vi "Begin.vi"() -> (1 "CameraDevRef":T1)   [LabVIEW 2011]
doc: "Called before other user functions, this VI is expected to open initial I/O refnums, load in file data, and do all program initialization. Notice that the <B>error out</B> terminal is simply used for data flow. Wiring it to other structures or subVIs ensures that this VI runs first."
uses:
  <vilib>/Rock Robotics/WPI/Camera/WPI_CameraDevRef.ctl
  <vilib>/Rock Robotics/SystemInterfaces/DIO/FPGA_DIOPWMChannel.ctl
  <vilib>/Rock Robotics/WPI/Joystick/WPI_JoystickDeviceEnum.ctl
  <vilib>/Rock Robotics/SystemInterfaces/AI/FPGA_AIChannel.ctl
  <vilib>/Rock Robotics/SystemInterfaces/DIO/FPGA_DIORelayChannel.ctl
  <vilib>/Rock Robotics/SystemInterfaces/DIO/FPGA_DIOChannel.ctl
  <vilib>/Rock Robotics/SystemInterfaces/AI/FPGA_AIGyroChannel.ctl
  <vilib>/Rock Robotics/WPI/MotorControl/WPI_MotorControlOpen Victor.vi
  <vilib>/Rock Robotics/WPI/MotorControl/WPI_MotorControlOpen Jaguar.vi
  Robot Global Data.vi
  <vilib>/Utility/file.llb/Read From Spreadsheet File (DBL).vi
  <vilib>/Rock Robotics/WPI/Relay/WPI_RelayDirection.ctl
  <vilib>/Rock Robotics/SystemInterfaces/Typedef/FPGA_TypedefDigitalModule.ctl
  <vilib>/Rock Robotics/WPI/Counter/WPI_CounterDigitalInputToDigitalSource.vi
  <vilib>/Rock Robotics/WPI/Encoder/WPI_EncoderType.ctl
  <vilib>/Rock Robotics/SystemInterfaces/Typedef/FPGA_TypedefAnalogModule.ctl
panel:
  out "Path and file":string
  in  "Balls In Robot At Start":dbl
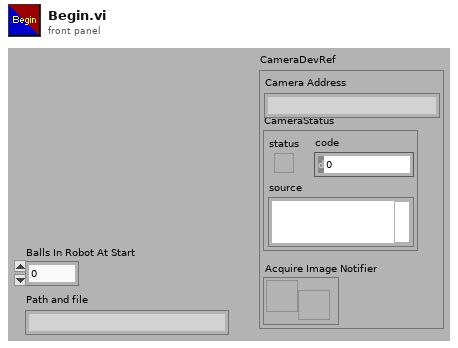
[diagram p1: front panel]
types:
  T1 = typedef "WPI_CameraDevRef.ctl" = cluster{"Camera Address":string, "CameraStatus":errorcluster, "Acquire Image Notifier":refnum<notifier>}
  T2 = typedef "FPGA_AIGyroChannel.ctl" = enum8{"AI 1", "AI 2", "Invalid"}
  T3 = typedef "FPGA_DIOChannel.ctl" = enum8{"DIO 1", "DIO 2", "DIO 3", "DIO 4", "DIO 5", "DIO 6", "DIO 7", "DIO 8", "DIO 9", "DIO 10", "DIO 11", "DIO 12", "DIO 13", "DIO 14", "Invalid"}
  T4 = typedef "FPGA_DIOPWMChannel.ctl" = enum8{"PWM 1", "PWM 2", "PWM 3", "PWM 4", "PWM 5", "PWM 6", "PWM 7", "PWM 8", "PWM 9", "PWM 10", "Invalid"}
  T5 = typedef "FPGA_DIORelayChannel.ctl" = enum8{"Relay 1", "Relay 2", "Relay 3", "Relay 4", "Relay 5", "Relay 6", "Relay 7", "Relay 8", "Invalid"}
  T6 = typedef "FPGA_AIChannel.ctl" = enum8{"AI 1", "AI 2", "AI 3", "AI 4", "AI 5", "AI 6", "AI 7", "AI 8", "Invalid"}
  T7 = typedef "WPI_JoystickDeviceEnum.ctl" = enum16{"USB 1", "USB 2", "USB 3", "USB 4", "Kinect 1", "Kinect 2"}
  T8 = typedef "WPI_CameraImageSize.ctl" = enum16{"640x480", "320x240", "160x120"}
  T9 = cluster{"fps":i32, "compression":i32, "Image Size":T8}
  T10 = typedef "WPI_MotorControlDeviceRef.ctl" = cluster{"DeviceStatus":errorcluster, "Type":enum16{"PWM", "CAN"}, "PWM":cluster{"Digital Module":T11, "PWM Channel":T4, "DeadBand":T12}, "CAN":cluster{"Device Number":u8, "Control Mode":T13, "Semaphore":T14, "Max Vout":dbl}, "Invert":bool, "TransformRef":T15, "InvTransformRef":T15}
  T11 = typedef "FPGA_TypedefDigitalModule.ctl" = enum16{"Digital Module 1", "Digital Module 2"}
  T12 = typedef "WPI_PWMDeadband.ctl" = cluster{"Name":string, "maxPositivePwm":i32, "minPositivePwm":i32, "centerPwm":i32, "maxNegativePwm":i32, "minNegativePwm":i32, "angularRange":u16}
  T13 = typedef "WPI_CANJaguar_ControlMode.ctl" = enum8{"Percent VBus", "Current", "Speed", "Position", "Voltage"}
  T14 = typedef "Semaphore RefNum" = refnum<k1>
  T15 = typedef "WPI_PWMTransform_ConPane.ctl" = refnum<vi>
  T16 = typedef "WPI_AnalogChannelDevRef.ctl" = cluster{"DevStatus":errorcluster, "Analog Module":T17, "Analog Channel":T6}
  T17 = typedef "FPGA_TypedefAnalogModule.ctl" = enum16{"Analog Module 1", "Analog Module 2"}
  T18 = typedef "WPI_ServoDeviceRef.ctl" = cluster{"DeviceStatus":errorcluster, "Digital Module":T11, "PWM Channel":T4, "DeadBand":T12}
  T19 = typedef "WPI_CameraWhite Balance Values.ctl" = enum16{"Auto", "Fixed indoor", "Fixed outdoor 1", "Fixed outdoor 2", "Fixed fluorescent 1", "Fixed fluorescent 2", "Hold current"}
  T20 = typedef "WPI_RelayDirection.ctl" = enum16{"Both directions", "Forward only", "Reverse only"}
  T21 = typedef "WPI_RelayDevRef.ctl" = cluster{"DevStatus":errorcluster, "Relay Channel":T5, "Digital Module":T11, "Relay Direction":T20}
  T22 = typedef "WPI_JoystickDevRef.ctl" = cluster{"Device":T7}
  T23 = typedef "WPI_CameraExposure Values.ctl" = enum16{"Auto", "Flicker-free 50 Hz", "Flicker-free 60 Hz", "Hold current"}
  T24 = typedef "WPI_EncoderType.ctl" = enum16{"1x", "2x", "4x"}
  T25 = typedef "WPI_DigitalInputDevRef.ctl" = cluster{"DevStatus":errorcluster, "DIO Channel":T3, "Digital Module":T11}
  T26 = typedef "FPGA_CounterEncoderSourceConvertionLVSourceType.ctl" = cluster{"DevStatus":errorcluster, "AnalogTriggerMode?":bool, "DigitalMode":cluster{"Digital Module":T11, "DIO Channel":T27}, "AnalogTriggerMode":cluster{"AnalogTriggerIndex":T28, "OutputType":T29}}
  T27 = typedef "FPGA_DIODigitalSourceChannel.ctl" = enum8{"DIO 1", "DIO 2", "DIO 3", "DIO 4", "DIO 5", "DIO 6", "DIO 7", "DIO 8", "DIO 9", "DIO 10", "DIO 11", "DIO 12", "DIO 13", "DIO 14", "Disabled"}
  T28 = typedef "FPGA_AnalogTriggerIndex.ctl" = enum8{"Trig 0", "Trig 1", "Trig 2", "Trig 3", "Trig 4", "Trig 5", "Trig 6", "Trig 7", "Invalid"}
  T29 = typedef "FPGA_AnalogTriggerOutType.ctl" = enum16{"InWindow", "TriggerState", "Rising", "Falling"}
  T30 = typedef "WPI_EncoderDevRef.ctl" = cluster{"DevStatus":errorcluster, "EncoderIndex":T31, "CounterIndex":T32, "DistancePerCount":dbl, "Decoding Type":T24}
  T31 = typedef "FPGA_EncoderIdx.ctl" = enum8{"Enc 0", "Enc 1", "Enc 2", "Enc 3", "Invalid"}
  T32 = typedef "FPGA_CounterCtrSystemIndex.ctl" = enum8{"Ctr 0", "Ctr 1", "Ctr 2", "Ctr 3", "Ctr 4", "Ctr 5", "Ctr 6", "Ctr 7", "Invalid"}
  T33 = typedef "WPI_GyroDevRef.ctl" = cluster{"DevStatus":errorcluster, "Analog Module":T17, "Analog Channel":T6, "Offset":dbl, "Gain (VoltsPerDegree/Second)":dbl}
  T34 = typedef "WPI_UltrasonicDeviceRef.ctl" = cluster{"DevStatus":errorcluster, "Ping Digital Module":T11, "Echo Digital Module":T11, "Ping Channel":T3, "Echo Channel":T3, "CntIndex":T32}
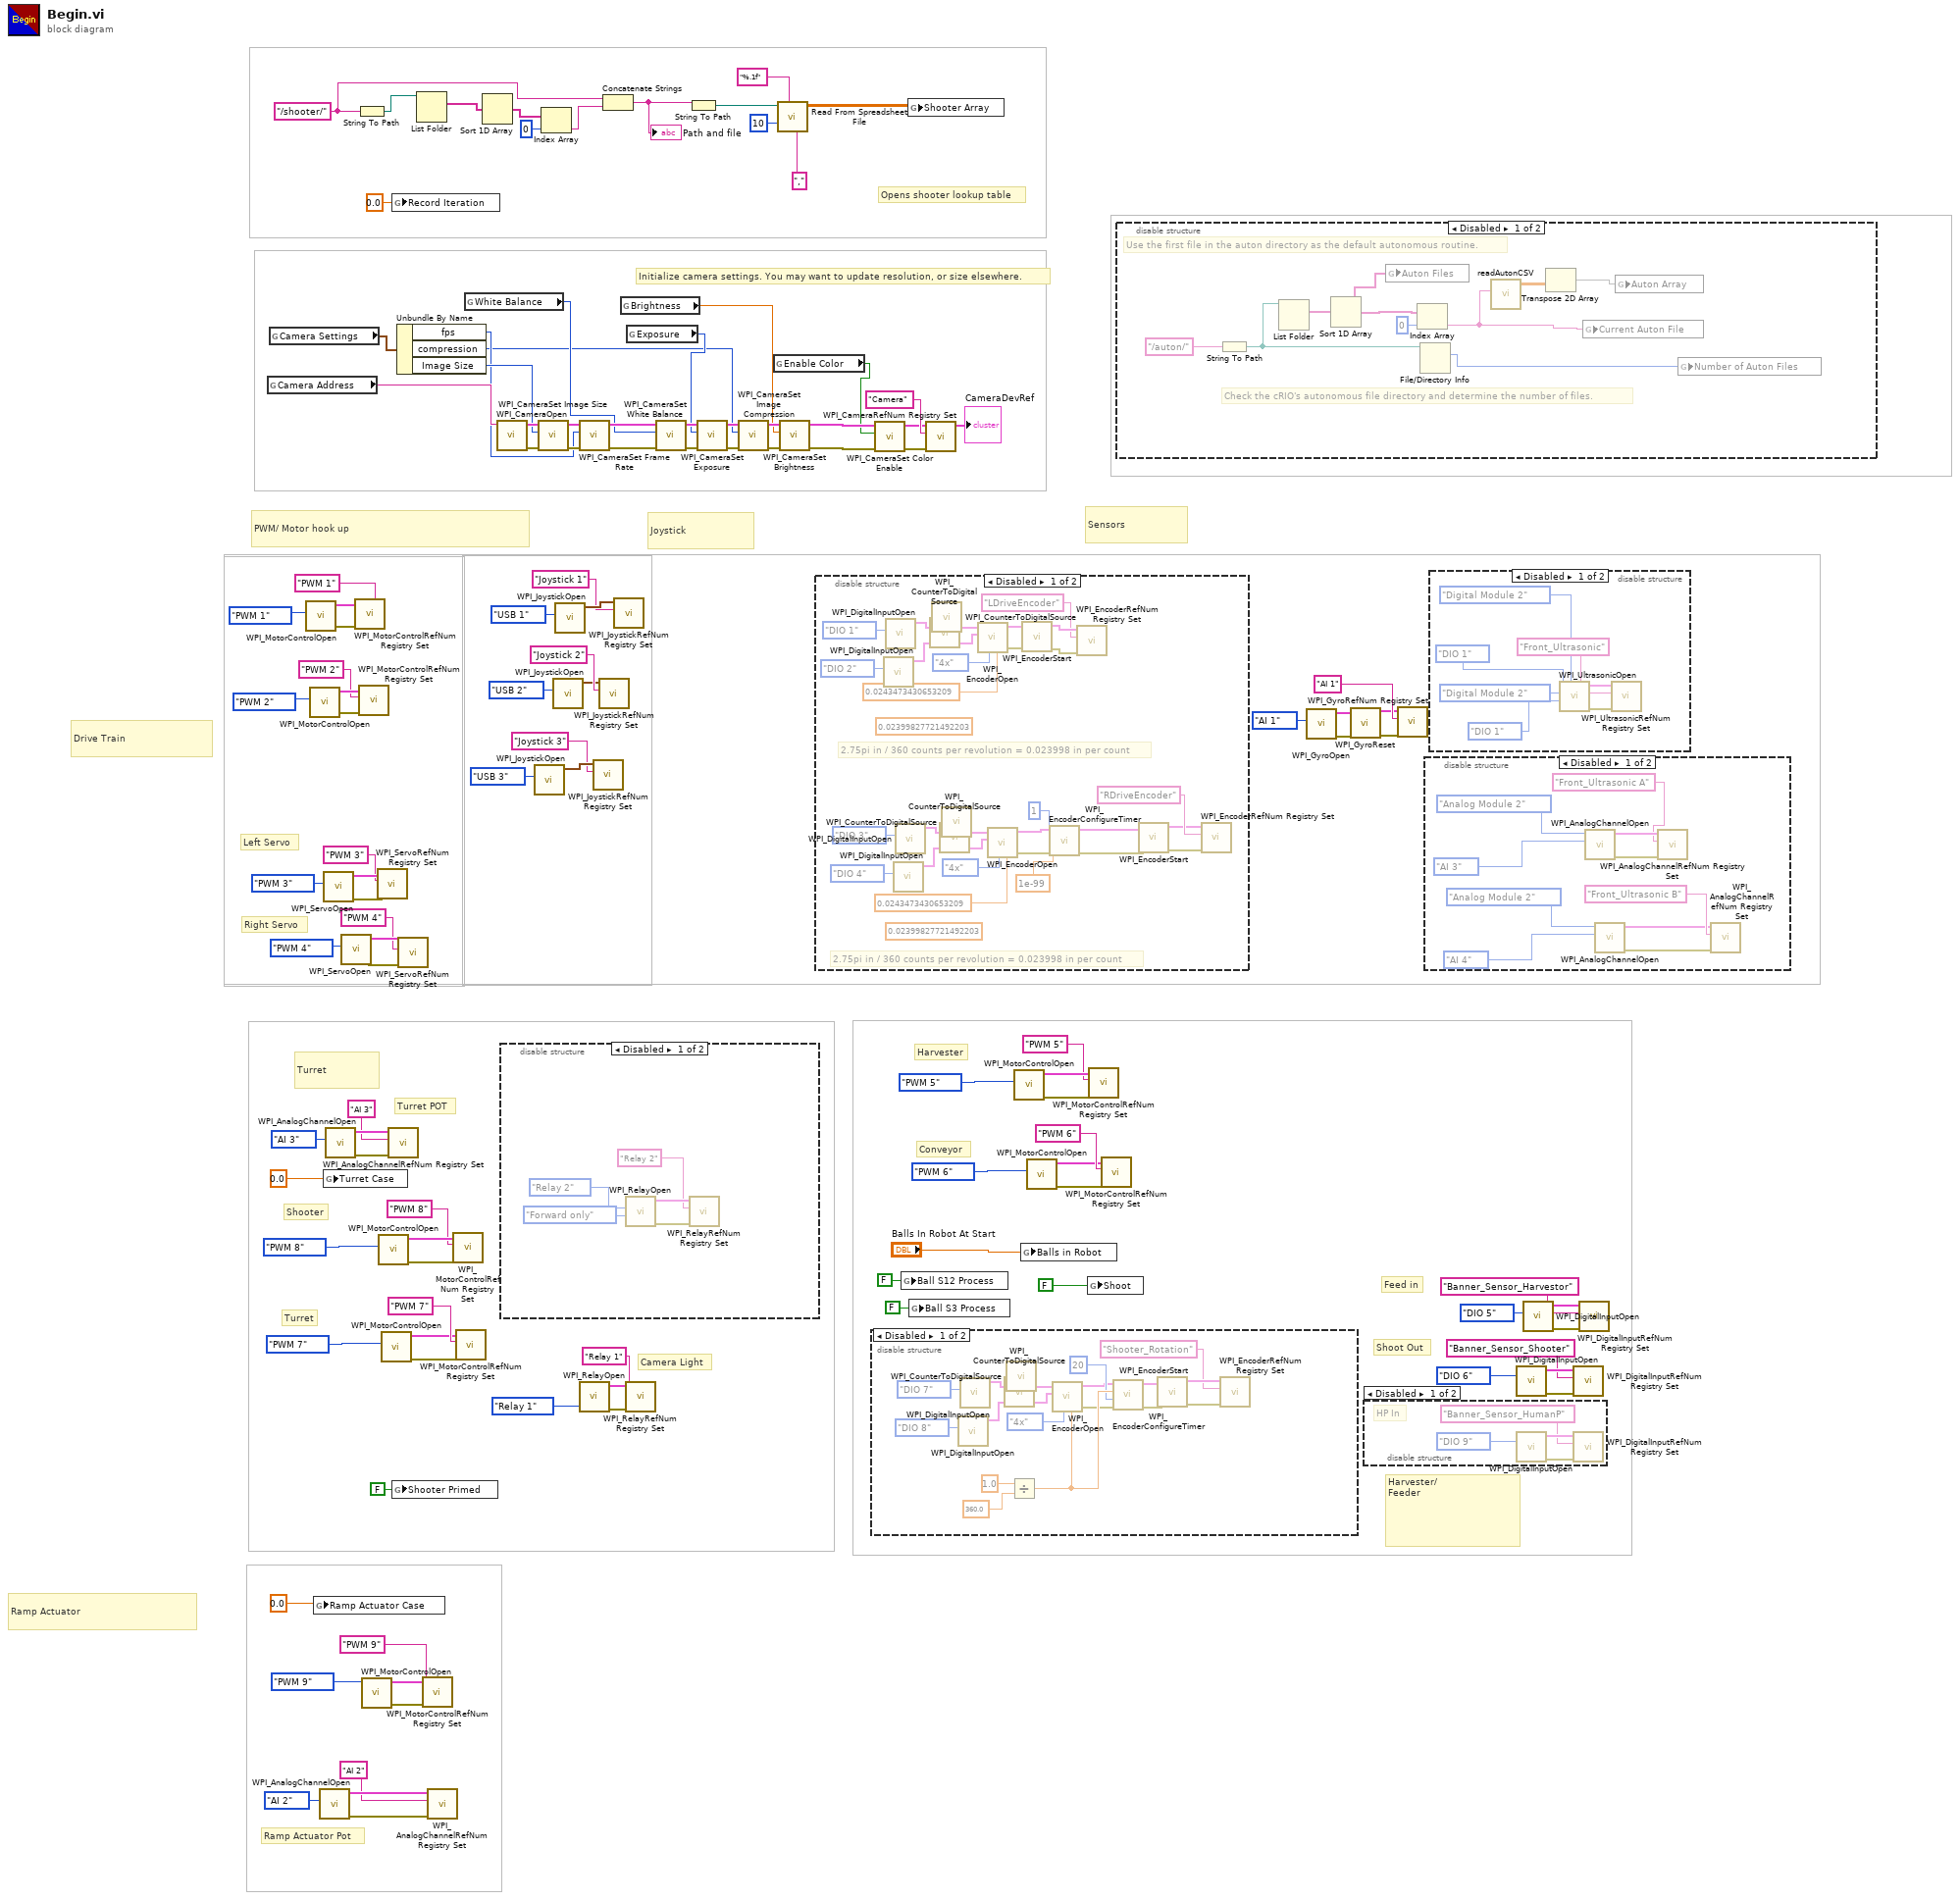
[diagram p0: block diagram]
diagram:
  w5 = "/shooter/" ("string")
  # "Opens shooter lookup table"
  # "Shoot Out"
  # "Feed in"
  # "Harvester"
  # "Conveyor"
  # "Shooter"
  # "Initialize camera settings. You may want to update resolution, or size elsewhere."
  # "Camera Light"
  # "Ramp Actuator Pot"
  # "Turret POT"
  # "Turret"
  # "Right Servo"
  # "Left Servo"
  # "Harvester/\nFeeder"
  # "Turret"
  # "Ramp Actuator"
  # "Drive Train"
  # "Sensors"
  # "Joystick"
  # "PWM/ Motor hook up"
  n1 = global read "Robot Global Data.vi" "Camera Address"() -> (w58:string)
  n2 = global read "Robot Global Data.vi" "Camera Settings"() -> (w57:T9)
  n3 = call-poly <vilib>:"WPI_MotorControlOpen.vi"("PWM Channel"=FPGA_DIOPWMChannel."PWM 1") -> ("error out"=w99:errorcluster, "MotorControlDeviceRef"=w101:T10)  [unwired: 9 in]
  n4 = call-poly <vilib>:"WPI_MotorControlOpen.vi"("PWM Channel"=FPGA_DIOPWMChannel."PWM 2") -> ("error out"=w97:errorcluster, "MotorControlDeviceRef"=w95:T10)  [unwired: 9 in]
  n5 = global write "Robot Global Data.vi" "Ramp Actuator Case"(0.0 ("Ramp Actuator Case")) -> ()
  n6 = call <vilib>:"WPI_AnalogChannelOpen.vi"("Analog Channel"=FPGA_AIChannel."AI 2") -> ("error out"=w83:errorcluster, "AIDeviceRef"=w84:T16)  [unwired: 9 in]
  n7 = call <vilib>:"WPI_ServoOpen.vi"("PWM Channel"=FPGA_DIOPWMChannel."PWM 3") -> ("error out"=w112:errorcluster, "ServoDeviceRef"=w117:T18)  [unwired: 9 in]
  n8 = global write "Robot Global Data.vi" "Turret Case"(0.0 ("Return To Home Case")) -> ()
  n9 = call <vilib>:"WPI_AnalogChannelOpen.vi"("Analog Channel"=FPGA_AIChannel."AI 3") -> ("error out"=w88:errorcluster, "AIDeviceRef"=w89:T16)  [unwired: 9 in]
  n10 = call <vilib>:"WPI_ServoOpen.vi"("PWM Channel"=FPGA_DIOPWMChannel."PWM 4") -> ("error out"=w111:errorcluster, "ServoDeviceRef"=w115:T18)  [unwired: 9 in]
  n11 = call <vilib>:"WPI_MotorControlRefNum Registry Set.vi"("error in (no error)"=w99, "refnum name"="PWM 1", "MotorControlDevRef"=w101) -> ()  [unwired: 7 in, 2 out]
  n12 = String To Path(string=w5) -> (path=w14:path)
  n13 = call <vilib>:"WPI_MotorControlRefNum Registry Set.vi"("error in (no error)"=w97, "refnum name"="PWM 2", "MotorControlDevRef"=w95) -> ()  [unwired: 7 in, 2 out]
  n14 = call-poly <vilib>:"WPI_MotorControlOpen.vi"("PWM Channel"=FPGA_DIOPWMChannel."PWM 9") -> ("error out"=w78:errorcluster, "MotorControlDeviceRef"=w79:T10)  [unwired: 9 in]
  n15 = call <vilib>:"WPI_ServoRefNum Registry Set.vi"("error in (no error)"=w112, "refnum name"="PWM 3", "ServoDeviceRef"=w117) -> ()  [unwired: 7 in, 2 out]
  n16 = call-poly <vilib>:"WPI_MotorControlOpen.vi"("PWM Channel"=FPGA_DIOPWMChannel."PWM 8") -> ("error out"=w41:errorcluster, "MotorControlDeviceRef"=w43:T10)  [unwired: 9 in]
  n17 = call-poly <vilib>:"WPI_MotorControlOpen.vi"("PWM Channel"=FPGA_DIOPWMChannel."PWM 7") -> ("error out"=w93:errorcluster, "MotorControlDeviceRef"=w91:T10)  [unwired: 9 in]
  n18 = call <vilib>:"WPI_AnalogChannelRefNum Registry Set.vi"("error in (no error)"=w88, "refnum name"="AI 3", "AIDeviceRef"=w89) -> ()  [unwired: 7 in, 2 out]
  n19 = global write "Robot Global Data.vi" "Record Iteration"(0.0 ("Record Iteration")) -> ()
  n20 = global write "Robot Global Data.vi" "Shooter Primed"(FALSE ("Ball S3 Process")) -> ()
  n21 = Unbundle By Name(w57) -> ("fps"=w55:i32, "compression"=w52:i32, "Image Size"=w56:T8)
  n22 = call <vilib>:"WPI_ServoRefNum Registry Set.vi"("error in (no error)"=w111, "refnum name"="PWM 4", "ServoDeviceRef"=w115) -> ()  [unwired: 7 in, 2 out]
  n23 = List Folder(path=w14) -> (filenames=w13:string[])  [unwired: 1 in, 5 out]
  n24 = call <vilib>:"WPI_MotorControlRefNum Registry Set.vi"("error in (no error)"=w78, "refnum name"="PWM 9", "MotorControlDevRef"=w79) -> ()  [unwired: 7 in, 2 out]
  n25 = call <vilib>:"WPI_AnalogChannelRefNum Registry Set.vi"("error in (no error)"=w83, "refnum name"="AI 2", "AIDeviceRef"=w84) -> ()  [unwired: 7 in, 2 out]
  n26 = call <vilib>:"WPI_MotorControlRefNum Registry Set.vi"("error in (no error)"=w41, "refnum name"="PWM 8", "MotorControlDevRef"=w43) -> ()  [unwired: 7 in, 2 out]
  n27 = call <vilib>:"WPI_MotorControlRefNum Registry Set.vi"("error in (no error)"=w93, "refnum name"="PWM 7", "MotorControlDevRef"=w91) -> ()  [unwired: 7 in, 2 out]
  n28 = global read "Robot Global Data.vi" "White Balance"() -> (w54:T19)
  n29 = Sort 1D Array(array=w13) -> (sorted array=w12:string[])
  n30 = call <vilib>:"WPI_CameraOpen.vi"("Camera Address"=w58) -> ("error out"=w64:errorcluster, "CameraDevRef"=w65:T1)  [unwired: 1 in, 8 out]
  n31 = disable-structure shown="Disabled" {
    frame Disabled {
      n32 = call <vilib>:"WPI_RelayOpen.vi"("Relay Direction"=WPI_RelayDirection."Forward only", "Relay Channel"=FPGA_DIORelayChannel."Relay 2") -> ("error out"=w122:errorcluster, "RelayDevRef"=w123:T21)  [unwired: 8 in]
      n33 = call <vilib>:"WPI_RelayRefNum Registry Set.vi"("error in (no error)"=w122, "refnum name"="Relay 2", "RelayDevRef"=w123) -> ()  [unwired: 7 in, 2 out]
    }
    frame Enabled {
    }
  }
  n34 = call <vilib>:"WPI_JoystickOpen.vi"("JoystickDevice"=WPI_JoystickDeviceEnum."USB 3") -> ("JoystickDevRef"=w104:T22)  [unwired: 10 in]
  n35 = call <vilib>:"WPI_CameraSet Image Size.vi"("error in (no error)"=w64, "Image Size"=w56, "CameraDevRef"=w65) -> ("error out"=w63:errorcluster, "CameraDevRef Out"=w66:T1)  [unwired: 7 out]
  n36 = Index Array(array=w12, index=0) -> (element=w4:string)
  n37 = call <vilib>:"WPI_JoystickOpen.vi"("JoystickDevice"=WPI_JoystickDeviceEnum."USB 2") -> ("JoystickDevRef"=w107:T22)  [unwired: 10 in]
  n38 = call <vilib>:"WPI_JoystickOpen.vi"("JoystickDevice"=WPI_JoystickDeviceEnum."USB 1") -> ("JoystickDevRef"=w110:T22)  [unwired: 10 in]
  n39 = call <vilib>:"WPI_CameraSet Frame Rate.vi"("error in (no error)"=w63, "Frame Rate (fps)"=w55, "CameraDevRef"=w66) -> ("error out"=w62:errorcluster, "CameraDevRef Out"=w68:T1)  [unwired: 7 out]
  n40 = call <vilib>:"WPI_RelayOpen.vi"("Relay Channel"=FPGA_DIORelayChannel."Relay 1") -> ("error out"=w75:errorcluster, "RelayDevRef"=w74:T21)  [unwired: 9 in]
  n41 = call <vilib>:"WPI_JoystickRefNum Registry Set.vi"("refnum name"="Joystick 3", "JoystickDevRef"=w104) -> ()  [unwired: 8 in, 2 out]
  n42 = call <vilib>:"WPI_JoystickRefNum Registry Set.vi"("refnum name"="Joystick 2", "JoystickDevRef"=w107) -> ()  [unwired: 8 in, 2 out]
  n43 = Concatenate Strings(w5, w4) -> (w7:string)
  "Path and file" <- w7
  n44 = call <vilib>:"WPI_JoystickRefNum Registry Set.vi"("refnum name"="Joystick 1", "JoystickDevRef"=w110) -> ()  [unwired: 8 in, 2 out]
  n45 = global read "Robot Global Data.vi" "Brightness"() -> (w51:dbl)
  n46 = call <vilib>:"WPI_RelayRefNum Registry Set.vi"("error in (no error)"=w75, "refnum name"="Relay 1", "RelayDevRef"=w74) -> ()  [unwired: 7 in, 2 out]
  n47 = global read "Robot Global Data.vi" "Exposure"() -> (w53:T23)
  n48 = call <vilib>:"WPI_CameraSet White Balance.vi"("error in (no error)"=w62, "White Balance"=w54, "CameraDevRef"=w68) -> ("error out"=w61:errorcluster, "CameraDevRef Out"=w67:T1)  [unwired: 7 out]
  n49 = String To Path(string=w7) -> (path=w6:path)
  n50 = call <vilib>:"WPI_CameraSet Exposure.vi"("error in (no error)"=w61, "Exposure"=w53, "CameraDevRef"=w67) -> ("error out"=w60:errorcluster, "CameraDevRef Out"=w70:T1)  [unwired: 7 out]
  n51 = call <vilib>:"WPI_CameraSet Image Compression.vi"("error in (no error)"=w60, "Compression"=w52, "CameraDevRef"=w70) -> ("error out"=w59:errorcluster, "CameraDevRef Out"=w69:T1)  [unwired: 7 out]
  n52 = global read "Robot Global Data.vi" "Enable Color"() -> (w46:bool)
  n53 = call-poly <vilib>:"Read From Spreadsheet File.vi"("delimiter (\\t)"="," ("delimiter (\\t)"), "format (%.3f)"="%.1f", "number of rows (all:-1)"=10, "file path (dialog if empty)"=w6) -> ("all rows"=w3:dbl[][])  [unwired: 1 in, 6 out]
  n54 = call <vilib>:"WPI_CameraSet Brightness.vi"("error in (no error)"=w59, "Brightness"=w51, "CameraDevRef"=w69) -> ("error out"=w49:errorcluster, "CameraDevRef Out"=w50:T1)  [unwired: 7 out]
  n55 = disable-structure shown="Disabled" {
    frame Disabled {
      (unwired) 0.02399827721492203 ("DistancePerCount")
      (unwired) 0.02399827721492203 ("DistancePerCount")
      # "2.75pi in / 360 counts per revolution = 0.023998 in per count"
      # "2.75pi in / 360 counts per revolution = 0.023998 in per count"
      n56 = call <vilib>:"WPI_DigitalInputOpen.vi"("DIO Channel"=FPGA_DIOChannel."DIO 2") -> ("DigitalInputDevRef"=w147:T25)  [unwired: 9 in, 1 out]
      n57 = call <vilib>:"WPI_DigitalInputOpen.vi"("DIO Channel"=FPGA_DIOChannel."DIO 1") -> ("DigitalInputDevRef"=w144:T25)  [unwired: 9 in, 1 out]
      n58 = call <vilib>:"WPI_DigitalInputOpen.vi"("DIO Channel"=FPGA_DIOChannel."DIO 4") -> ("DigitalInputDevRef"=w138:T25)  [unwired: 9 in, 1 out]
      n59 = call <vilib>:"WPI_DigitalInputOpen.vi"("DIO Channel"=FPGA_DIOChannel."DIO 3") -> ("DigitalInputDevRef"=w141:T25)  [unwired: 9 in, 1 out]
      n60 = call-poly <vilib>:"WPI_CounterToDigitalSource.vi"("DigitalInputDevRef"=w147) -> ("Digital Source"=w148:T26)  [unwired: 6 in]
      n61 = call-poly <vilib>:"WPI_CounterToDigitalSource.vi"("DigitalInputDevRef"=w144) -> ("Digital Source"=w143:T26)  [unwired: 6 in]
      n62 = call-poly <vilib>:"WPI_CounterToDigitalSource.vi"("DigitalInputDevRef"=w138) -> ("Digital Source"=w137:T26)  [unwired: 6 in]
      n63 = call-poly <vilib>:"WPI_CounterToDigitalSource.vi"("DigitalInputDevRef"=w141) -> ("Digital Source"=w142:T26)  [unwired: 6 in]
      n64 = call <vilib>:"WPI_EncoderOpen.vi"("DistancePerCount"=0.0243473430653209, "Decoding Type"=WPI_EncoderType."4x", "BSource"=w148, "ASource"=w143) -> ("error out"=w150:errorcluster, "EncoderDevRef"=w151:T30)  [unwired: 6 in]
      n65 = call <vilib>:"WPI_EncoderOpen.vi"("DistancePerCount"=0.0243473430653209, "Decoding Type"=WPI_EncoderType."4x", "BSource"=w137, "ASource"=w142) -> ("error out"=w134:errorcluster, "EncoderDevRef"=w133:T30)  [unwired: 6 in]
      n66 = call <vilib>:"WPI_EncoderStart.vi"("error in (no error)"=w150, "EncoderDevRef"=w151) -> ("error out"=w153:errorcluster, "EncoderDevRef"=w152:T30)  [unwired: 8 in]
      n67 = call <vilib>:"WPI_EncoderConfigureTimer.vi"("error in (no error)"=w134, "Number Samples to Average"=u8 1, "Minimum Rate"=1e-99, "EncoderDevRef"=w133) -> ("error out"=w129:errorcluster, "EncoderDevRef"=w130:T30)  [unwired: 6 in]
      n68 = call <vilib>:"WPI_EncoderRefNum Registry Set.vi"("error in (no error)"=w153, "refnum name"="LDriveEncoder", "EncoderDevRef"=w152) -> ()  [unwired: 7 in, 2 out]
      n69 = call <vilib>:"WPI_EncoderStart.vi"("error in (no error)"=w129, "EncoderDevRef"=w130) -> ("error out"=w127:errorcluster, "EncoderDevRef"=w128:T30)  [unwired: 8 in]
      n70 = call <vilib>:"WPI_EncoderRefNum Registry Set.vi"("error in (no error)"=w127, "refnum name"="RDriveEncoder", "EncoderDevRef"=w128) -> ()  [unwired: 7 in, 2 out]
    }
    frame Enabled {
    }
  }
  n71 = disable-structure shown="Disabled" {
    frame Disabled {
      n72 = call <vilib>:"WPI_DigitalInputOpen.vi"("DIO Channel"=FPGA_DIOChannel."DIO 8") -> ("DigitalInputDevRef"=w158:T25)  [unwired: 9 in, 1 out]
      n73 = call <vilib>:"WPI_DigitalInputOpen.vi"("DIO Channel"=FPGA_DIOChannel."DIO 7") -> ("DigitalInputDevRef"=w155:T25)  [unwired: 9 in, 1 out]
      n74 = call-poly <vilib>:"WPI_CounterToDigitalSource.vi"("DigitalInputDevRef"=w158) -> ("Digital Source"=w159:T26)  [unwired: 6 in]
      n75 = call-poly <vilib>:"WPI_CounterToDigitalSource.vi"("DigitalInputDevRef"=w155) -> ("Digital Source"=w154:T26)  [unwired: 6 in]
      n76 = Divide(x=1.0, y=360.0) -> (x/y=w171:dbl)
      n77 = call <vilib>:"WPI_EncoderOpen.vi"("DistancePerCount"=w171, "Decoding Type"=WPI_EncoderType."4x", "BSource"=w159, "ASource"=w154) -> ("error out"=w162:errorcluster, "EncoderDevRef"=w163:T30)  [unwired: 6 in]
      n78 = call <vilib>:"WPI_EncoderConfigureTimer.vi"("error in (no error)"=w162, "Number Samples to Average"=u8 20, "Minimum Rate"=w171, "EncoderDevRef"=w163) -> ("error out"=w166:errorcluster, "EncoderDevRef"=w165:T30)  [unwired: 6 in]
      n79 = call <vilib>:"WPI_EncoderStart.vi"("error in (no error)"=w166, "EncoderDevRef"=w165) -> ("error out"=w168:errorcluster, "EncoderDevRef"=w167:T30)  [unwired: 8 in]
      n80 = call <vilib>:"WPI_EncoderRefNum Registry Set.vi"("error in (no error)"=w168, "refnum name"="Shooter_Rotation", "EncoderDevRef"=w167) -> ()  [unwired: 7 in, 2 out]
    }
    frame Enabled {
    }
  }
  n81 = call <vilib>:"WPI_CameraSet Color Enable.vi"("error in (no error)"=w49, "Color Enabled"=w46, "CameraDevRef"=w50) -> ("error out"=w47:errorcluster, "CameraDevRef Out"=w48:T1)  [unwired: 7 in]
  n82 = global write "Robot Global Data.vi" "Ball S12 Process"(FALSE ("Ball S12 Process")) -> ()
  n83 = global write "Robot Global Data.vi" "Shooter Array"(w3) -> ()
  n84 = global write "Robot Global Data.vi" "Ball S3 Process"(FALSE ("Ball S3 Process")) -> ()
  n85 = call <vilib>:"WPI_CameraRefNum Registry Set.vi"("error in (no error)"=w47, "refnum name"="Camera", "CameraDevRef"=w48) -> ("CameraDevRef"=→"CameraDevRef":T1)  [unwired: 8 out]
  n86 = call-poly <vilib>:"WPI_MotorControlOpen.vi"("PWM Channel"=FPGA_DIOPWMChannel."PWM 5") -> ("error out"=w37:errorcluster, "MotorControlDeviceRef"=w39:T10)  [unwired: 9 in]
  n87 = global write "Robot Global Data.vi" "Balls in Robot"("Balls In Robot At Start") -> ()
  n88 = call-poly <vilib>:"WPI_MotorControlOpen.vi"("PWM Channel"=FPGA_DIOPWMChannel."PWM 6") -> ("error out"=w36:errorcluster, "MotorControlDeviceRef"=w34:T10)  [unwired: 9 in]
  n89 = global write "Robot Global Data.vi" "Shoot"(FALSE ("Ball S12 Process")) -> ()
  n90 = call <vilib>:"WPI_MotorControlRefNum Registry Set.vi"("error in (no error)"=w37, "refnum name"="PWM 5", "MotorControlDevRef"=w39) -> ()  [unwired: 7 in, 2 out]
  n91 = call <vilib>:"WPI_MotorControlRefNum Registry Set.vi"("error in (no error)"=w36, "refnum name"="PWM 6", "MotorControlDevRef"=w34) -> ()  [unwired: 7 in, 2 out]
  n92 = disable-structure shown="Disabled" {
    frame Disabled {
      # "Check the cRIO's autonomous file directory and determine the number of files."
      # "Use the first file in the auton directory as the default autonomous routine."
      n93 = String To Path(string="/auton/") -> (path=w179:path)
      n94 = List Folder(path=w179) -> (filenames=w178:string[])  [unwired: 1 in, 5 out]
      n95 = Sort 1D Array(array=w178) -> (sorted array=w174:string[])
      n96 = global write "Robot Global Data.vi" "Auton Files"(w174) -> ()
      n97 = Index Array(array=w174, index=0) -> (element=w175:string)
      n98 = File/Directory Info(path=w179) -> (size=w176:i64)  [unwired: 1 in, 6 out]
      n99 = call "readAutonCSV.vi"("AutonFile"=w175) -> ("AutonArray"=w173:dbl[][])  [unwired: 7 in]
      n100 = Transpose 2D Array(2D array=w173) -> (transposed array=w172:dbl[][])
      n101 = global write "Robot Global Data.vi" "Current Auton File"(w175) -> ()
      n102 = global write "Robot Global Data.vi" "Auton Array"(w172) -> ()
      n103 = global write "Robot Global Data.vi" "Number of Auton Files"(w176) -> ()
    }
    frame Enabled {
    }
  }
  n104 = call <vilib>:"WPI_GyroOpen.vi"("Analog Channel"=FPGA_AIGyroChannel."AI 1") -> ("error out"=w17:errorcluster, "GyroDevRef"=w18:T33)  [unwired: 8 in, 1 out]
  n105 = call <vilib>:"WPI_GyroReset.vi"("error in (no error)"=w17, "GyroDevRef"=w18) -> ("error out"=w16:errorcluster, "GyroDevRef"=w15:T33)  [unwired: 8 in]
  n106 = disable-structure shown="Disabled" {
    frame Disabled {
      # "HP In"
      n107 = call <vilib>:"WPI_DigitalInputOpen.vi"("DIO Channel"=FPGA_DIOChannel."DIO 9") -> ("error out"=w183:errorcluster, "DigitalInputDevRef"=w182:T25)  [unwired: 9 in]
      n108 = call <vilib>:"WPI_DigitalInputRefNum Registry Set.vi"("error in (no error)"=w183, "refnum name"="Banner_Sensor_HumanP", "DigitalInputDevRef"=w182) -> ()  [unwired: 7 in, 2 out]
    }
    frame Enabled {
    }
  }
  n109 = call <vilib>:"WPI_GyroRefNum Registry Set.vi"("error in (no error)"=w16, "refnum name"="AI 1", "GyroDevRef"=w15) -> ()  [unwired: 7 in, 2 out]
  n110 = disable-structure shown="Disabled" {
    frame Disabled {
      n111 = call <vilib>:"WPI_AnalogChannelOpen.vi"("Analog Channel"=FPGA_AIChannel."AI 3", "Analog Module (Module 1)"=FPGA_TypedefAnalogModule."Analog Module 2") -> ("error out"=w190:errorcluster, "AIDeviceRef"=w189:T16)  [unwired: 8 in]
      n112 = call <vilib>:"WPI_AnalogChannelOpen.vi"("Analog Channel"=FPGA_AIChannel."AI 4", "Analog Module (Module 1)"=FPGA_TypedefAnalogModule."Analog Module 2") -> ("error out"=w185:errorcluster, "AIDeviceRef"=w186:T16)  [unwired: 8 in]
      n113 = call <vilib>:"WPI_AnalogChannelRefNum Registry Set.vi"("error in (no error)"=w190, "refnum name"="Front_Ultrasonic A", "AIDeviceRef"=w189) -> ()  [unwired: 7 in, 2 out]
      n114 = call <vilib>:"WPI_AnalogChannelRefNum Registry Set.vi"("error in (no error)"=w185, "refnum name"="Front_Ultrasonic B", "AIDeviceRef"=w186) -> ()  [unwired: 7 in, 2 out]
    }
    frame Enabled {
    }
  }
  n115 = disable-structure shown="Disabled" {
    frame Disabled {
      n116 = call <vilib>:"WPI_UltrasonicOpen.vi"("Ping Digital Module (Module 1)"=FPGA_TypedefDigitalModule."Digital Module 2", "Echo DIO Channel"=FPGA_DIOChannel."DIO 1", "Echo Digital Module (Module 1)"=FPGA_TypedefDigitalModule."Digital Module 2", "Ping DIO Channel"=FPGA_DIOChannel."DIO 1") -> ("error out"=w201:errorcluster, "UltrasonicDevRef"=w200:T34)  [unwired: 6 in]
      n117 = call <vilib>:"WPI_UltrasonicRefNum Registry Set.vi"("error in (no error)"=w201, "refnum name"="Front_Ultrasonic", "UltrasonicDevRef"=w200) -> ()  [unwired: 7 in, 2 out]
    }
    frame Enabled {
    }
  }
  n118 = call <vilib>:"WPI_DigitalInputOpen.vi"("DIO Channel"=FPGA_DIOChannel."DIO 6") -> ("error out"=w27:errorcluster, "DigitalInputDevRef"=w26:T25)  [unwired: 9 in]
  n119 = call <vilib>:"WPI_DigitalInputOpen.vi"("DIO Channel"=FPGA_DIOChannel."DIO 5") -> ("error out"=w30:errorcluster, "DigitalInputDevRef"=w29:T25)  [unwired: 9 in]
  n120 = call <vilib>:"WPI_DigitalInputRefNum Registry Set.vi"("error in (no error)"=w27, "refnum name"="Banner_Sensor_Shooter", "DigitalInputDevRef"=w26) -> ()  [unwired: 7 in, 2 out]
  n121 = call <vilib>:"WPI_DigitalInputRefNum Registry Set.vi"("error in (no error)"=w30, "refnum name"="Banner_Sensor_Harvestor", "DigitalInputDevRef"=w29) -> ()  [unwired: 7 in, 2 out]
